vi "Refresh Constants.vi"() -> ()   [LabVIEW 2020, in "Ballard ARINC 429 System Explorer.lvlib" / "Implementation.lvlib"]
uses:
  Implementation.lvlib
panel:
  in  "Timestamp":string="Timestamp"
  in  "Unit":string="Unit"
  in  "Scale Offset":string="Scale Offset"
  in  "Scale Factor":string="Scale Factor"
  in  "Signed":string="Signed"
  in  "Size":string="Size"
  in  "Start Index":string="Start Index"
  in  "Default Value":string="Default Value"
  in  "Encoding":string="Encoding"
  in  "Transfer Type":string="Transfer Type"
  in  "SDI Value":string="SDI Value"
  in  "SDI Enabled":string="SDI Enabled"
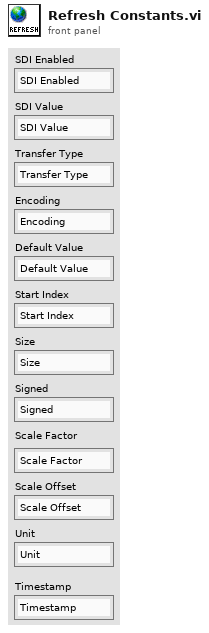
[diagram p1: front panel]
diagram:
